vi "filterWheelThorlabsMove.vi"(1 "position":u8) -> ()   [LabVIEW 2017]
uses:
  globalDevices.vi
panel:
  out "concatenated string":string
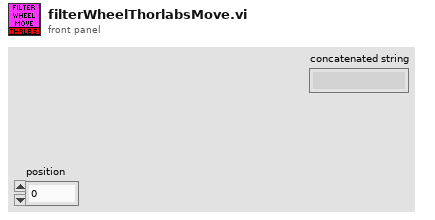
[diagram p1: front panel]
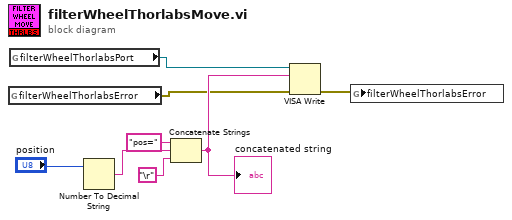
[diagram p0: block diagram]
diagram:
  n1 = global read "globalDevices.vi" "filterWheelThorlabsError"() -> (w2:errorcluster)
  n2 = global read "globalDevices.vi" "filterWheelThorlabsPort"() -> (w3:refnum<visa-resource-name>)
  n3 = Number To Decimal String(number="position") -> (decimal integer string=w7:string)  [unwired: 1 in]
  n4 = Concatenate Strings("pos=" ("string"), w7, "\r") -> (w4:string)
  "concatenated string" <- w4
  n5 = VISA Write(VISA resource name=w3, write buffer=w4, error in (no error)=w2) -> (error out=w1:errorcluster)  [unwired: 2 out]
  n6 = global write "globalDevices.vi" "filterWheelThorlabsError"(w1) -> ()
